vi "Stop Target.vi"(8 "error in":errorcluster, 10 "Target Ident":string, 11 "Host Measure and Stimulus Subsystems in":refnum<class "Host Measure and Stimulus Subsystems.lvclass">) -> (0 "error out":errorcluster, 3 "Host Measure and Stimulus Subsystems out":refnum<class "Host Measure and Stimulus Subsystems.lvclass">)   [LabVIEW 2023, in "HAL GOOP4.lvlib" / "Host Measure and Stimulus Subsystems.lvclass"]
uses:
  Host Measure and Stimulus Subsystems.lvclass
  Host Measure and Stimulus Subsystems.lvclass/Host Measure and Stimulus Subsystems.ctl
  Virtual Instrument Base/Virt Instr Base.lvclass
  <vilib>/Utility/error.llb/Error Cluster From Error Code.vi
  <vilib>/ErrorRing/Error Ring.xnode
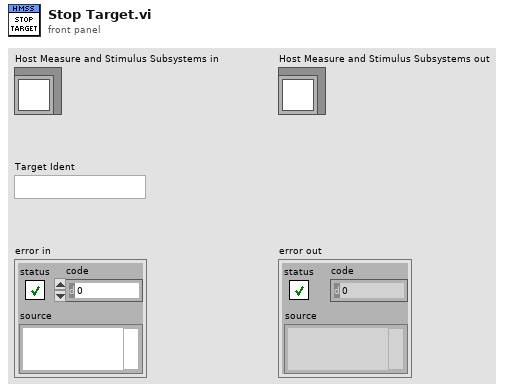
[diagram p1: front panel]
types:
  T1 = map{string, refnum<class "Virt Instr Base.lvclass">}
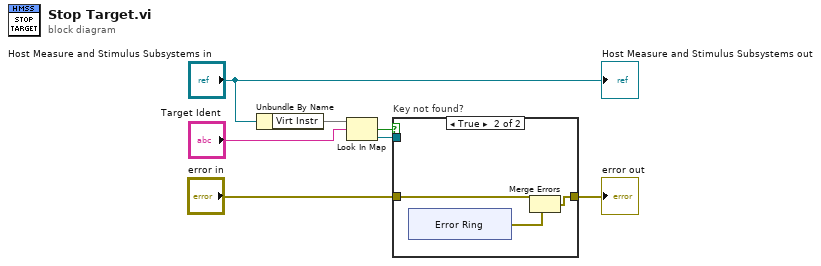
[diagram p0: block diagram]
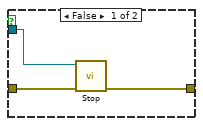
[diagram p2: hidden frame]
diagram:
  n1 = Unbundle By Name("Host Measure and Stimulus Subsystems in") -> ("Virt Instr"=w6:T1)
  n2 = Look In Map(map=w6, key="Target Ident") -> (key not found?=w4:bool, value=w3:refnum<class "Virt Instr Base.lvclass">)  [unwired: 1 in]
  n3 = case "Key not found?" shown="True" w4 {
    tunnel: w3 -> [w9 _]
    tunnel: "error in" -> [w8 w11]
    tunnel: [w10 w13] -> w2
    frame False {
      n4 = call "Stop.vi"("error in (no error)"=w8, "Virt Instr Base in"=w9) -> ("error out"=w10:errorcluster)  [unwired: 8 in, 1 out]
    }
    frame True {
      n5 = xnode "Error Ring"() -> ("error out"=w12:errorcluster)
      n6 = Merge Errors(w11, w12) -> (w13:errorcluster)
    }
  }
  "error out" <- w2
  "Host Measure and Stimulus Subsystems out" <- "Host Measure and Stimulus Subsystems in"
